vi "Agilent Counter VI.vi"() -> ()   [LabVIEW 2011]
doc: "This example shows how to acquire frequency through sending a trigger."
uses:
  <instrlib>/Agilent 53147/Public/Configure/Configure Measurement (Frequency).vi
  <vilib>/Utility/file.llb/Write To Spreadsheet File (DBL).vi
  <instrlib>/Agilent 53147/Agilent 53147.lvlib
panel:
  in  "export path":path=path "C:/Users/VGroup/Desktop/data/test_agilent2.txt"
  out "appended array":dbl[](array[numeric])=[23.0, 140618.0, 164949.0, 12000000000.0]
  out "date number":i32=140618
  out "time number":i32=164949
  in  "time format string 2":string="%H%M%S" caption="time format string2 (%d%m%y-%H%M%S)"
  out "time string":string="164949"
  out "date string":string="140618"
  in  "time format string":string="%y%m%d" caption="time format string1 (%d%m%y-%H%M%S)"
  in  "seconds to wait":u32=1
  in  "stop":bool
  in  "Channel (2:Channel 2)":i32(ring)=2 items=["Channel 1"=1, "Channel 2"=2]
  in  "Timeout (10000 ms)":u32=10000
  out "Frequency Measurement":dbl=12000000000.0
  in  "VISA resource name":refnum<visa-resource-name>="GPIB0::19::INSTR"
  # "(c) 2010 <National Instruments>.  ALL RIGHTS RESERVED."
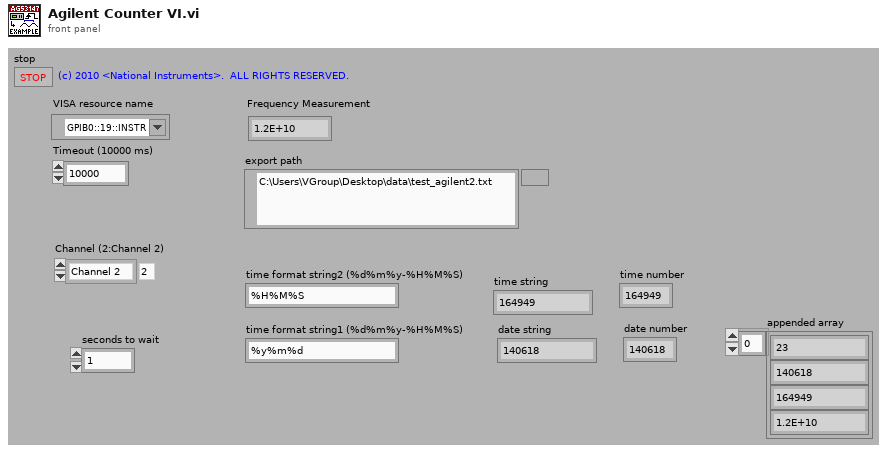
[diagram p1: front panel]
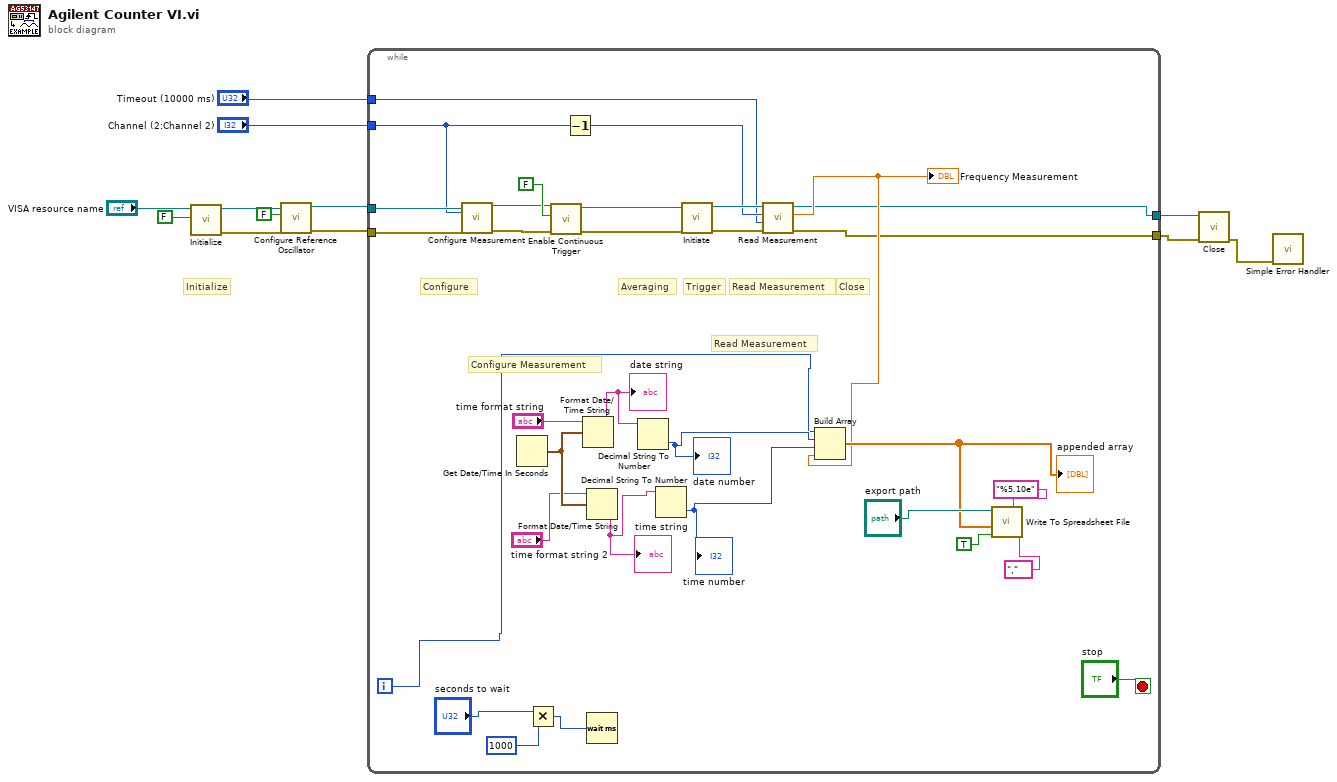
[diagram p0: block diagram]
diagram:
  # "Initialize"
  n1 = call <instrlib>:"Initialize.vi"("ID Query (True)"=FALSE, "VISA resource name"="VISA resource name") -> ("error out"=w5:errorcluster, "VISA resource name out"=w3:refnum<visa-resource-name>)  [unwired: 8 in]
  n2 = call <instrlib>:"Configure Reference Oscillator.vi"("error in (no error)"=w5, "Source (T: Internal)"=FALSE, "VISA resource name"=w3) -> ("error out"=w4:errorcluster, "VISA resource name out"=w2:refnum<visa-resource-name>)  [unwired: 7 in]
  n3 = while {
    tunnel: w2 -> [w44]
    tunnel: w4 -> [w43]
    tunnel: "Timeout (10000 ms)" -> [w36]
    tunnel: "Channel (2:Channel 2)" -> [w35]
    tunnel: [w17] -> w8
    tunnel: [w16] -> w7
    i -> [w19]
    stop <- "stop" stop-if-true
    # "Read Measurement"
    # "Configure Measurement"
    # "Trigger"
    # "Close"
    # "Read Measurement"
    # "Averaging"
    # "Configure"
    n4 = call-poly <instrlib>:"Configure Measurement.vi"("VISA resource name"=w44, "Channel (2:Channel 2)"=w35, "error in (no error)"=w43) -> ("VISA resource name out"=w37:refnum<visa-resource-name>, "error out"=w38:errorcluster)  [unwired: 11 in]
    n5 = Get Date/Time In Seconds() -> (seconds since 1Jan1904=w30:timestamp)
    n6 = Multiply(x="seconds to wait", y=u32 1000) -> (x*y=w13:u32)
    n7 = call <instrlib>:"Enable Continuous Trigger.vi"("error in (no error)"=w38, "Enable Continuous Trigger (T: Enable)"=FALSE ("Enable Continous Trigger (T: Enable)"), "VISA resource name"=w37) -> ("error out"=w33:errorcluster, "VISA resource name out"=w34:refnum<visa-resource-name>)  [unwired: 7 in]
    n8 = Decrement(x=w35) -> (x-1=w40:i32)
    n9 = Format Date/Time String(time format string (%c)="time format string", seconds (now)=w30) -> (date/time string=w27:string)  [unwired: 1 in]
    "date string" <- w27
    n10 = Format Date/Time String(time format string (%c)="time format string 2", seconds (now)=w30) -> (date/time string=w28:string)  [unwired: 1 in]
    "time string" <- w28
    n11 = Wait (ms)(milliseconds to wait=w13) -> ()  [unwired: 1 out]
    n12 = Decimal String To Number(string=w27) -> (number=w26:i32)  [unwired: 2 in, 1 out]
    "date number" <- w26
    n13 = Decimal String To Number(string=w28) -> (number=w25:i32)  [unwired: 2 in, 1 out]
    "time number" <- w25
    n14 = call <instrlib>:"Initiate.vi"("error in (no error)"=w33, "VISA resource name"=w34) -> ("error out"=w41:errorcluster, "VISA resource name out"=w42:refnum<visa-resource-name>)  [unwired: 8 in]
    n15 = call <instrlib>:"Read Measurement.vi"("error in (no error)"=w41, "Timeout (10000 ms)"=w36, "Measurement Function (0: Frequency)"=w40, "VISA resource name"=w42) -> ("error out"=w16:errorcluster, "Measurement"=w18:dbl, "VISA resource name out"=w17:refnum<visa-resource-name>)  [unwired: 5 in]
    "Frequency Measurement" <- w18
    n16 = Build Array(w19, w26, w25, w18) -> (w21:dbl[])
    "appended array" <- w21
    n17 = call-poly <vilib>:"Write To Spreadsheet File.vi"("delimiter (\\t)"="," ("delimiter (Tab)"), "format (%.3f)"="%5.10e", "append to file? (new file:F)"=TRUE ("transpose? (no:F)"), "1D data"=w21, "file path (dialog if empty)"="export path") -> ()  [unwired: 3 in, 1 out]
  }
  n18 = call <instrlib>:"Close.vi"("error in (no error)"=w7, "VISA resource name"=w8) -> ("error out"=w6:errorcluster)  [unwired: 9 in]
  n19 = call <vilib>:"Simple Error Handler.vi"("error in (no error)"=w6) -> ()  [unwired: 4 in, 5 out]
